vi "Get as DBL Array.vi"(8 "error in (no error)":errorcluster, 11 "JSON Array in":refnum<class "JSON Value.lvclass">) -> (0 "error out":errorcluster, 2 "Array of numbers":dbl[](array[numeric]), 3 "JSON Array out":refnum<class "JSON Value.lvclass">)   [LabVIEW 2011, in "JSON Array.lvclass"]
uses:
  JSON Array.lvclass
  JSON Value/JSON Value.lvclass
  JSON Scalar/JSON Scalar.lvclass
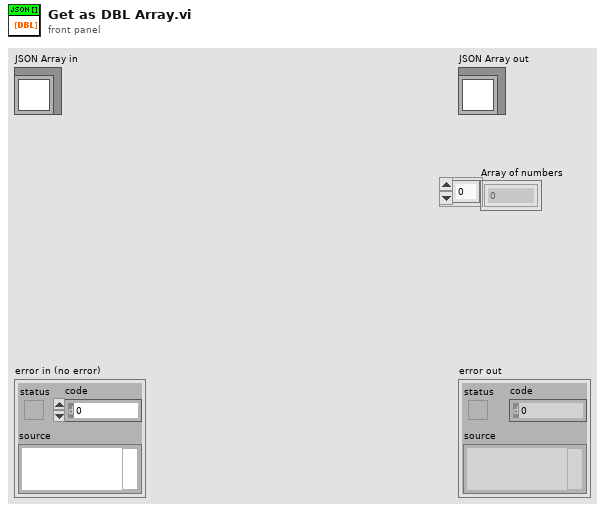
[diagram p1: front panel]
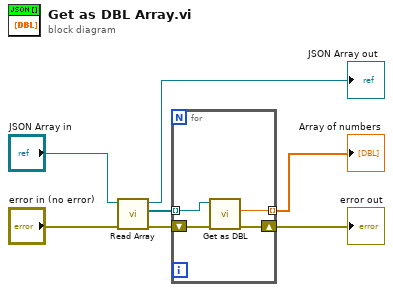
[diagram p0: block diagram]
diagram:
  n1 = call-dynamic "Read Array.vi"("error in (no error)"="error in (no error)", "JSON Value In"="JSON Array in") -> ("error out"=w2:errorcluster, "Array"=w3:refnum<class "JSON Value.lvclass">[], "JSON Value Out"=→"JSON Array out":refnum<class "JSON Value.lvclass">)  [unwired: 7 in]
  n2 = for {
    tunnel: w3 -> [w9] mode=indexing
    shift-right: [w11] -> w6
    shift-left: w2 -> [w8]
    tunnel: [w10] -> w1 mode=indexing
    n3 = call "Get as DBL.vi"("error in (no error)"=w8, "JSON Value in"=w9) -> ("error out"=w11:errorcluster, "Number"=w10:dbl)  [unwired: 7 in, 1 out]
  }
  "error out" <- w6
  "Array of numbers" <- w1
